vi "UI.KeyCheck.vi"(7 "baud rate (9600)":u32=9600 caption="波特率(9600)", 8 "error in (no error)":errorcluster caption="错误输入（无错误）", 9 "KeyDelay(s)":dbl=8.0 format="%#_2g", 10 "VISA resource name":refnum<visa-resource-name> caption="Serial Port", 11 "KeyList":path) -> (0 "error out":errorcluster caption="错误输出", 3 "Result?":bool, 6 "Test Process":string="Descripte test process.")   [LabVIEW 2012, in "Lib_UEL.ATE.lvlib" / "Lib_App.lvlib"]
uses:
  Lib_App.lvlib
  <vilib>/Utility/config.llb/Read Key (String).vi
  <vilib>/Instr/_visa.llb/VISA Configure Serial Port (Instr).vi
  <vilib>/Utility/config.llb/NI_LVConfig.lvlib
panel:
  in  "para":enum32{"para"}(tab)
  in  "计时":bool
  in  "RS232_ON?":bool
  in  "重置计时":bool=TRUE caption="重置"
  out "KeyCheckOK?":bool[](array[boolean])
  in  "停止":bool
  out "KeyValue":string[](array[string])
  out "Key Frame Check":string
  out "KEY10":bool caption="KEY1"
  out "KEY9":bool caption="KEY1"
  out "KEY8":bool caption="KEY1"
  out "KEY7":bool caption="KEY1"
  out "KEY6":bool caption="KEY1"
  out "KEY5":bool caption="KEY1"
  out "KEY4":bool caption="KEY1"
  out "KEY3":bool caption="KEY1"
  out "KEY2":bool caption="KEY1"
  out "KEY1":bool
  out "KeyTime":dbl format="%05.2f"
  out "Key Frame":string
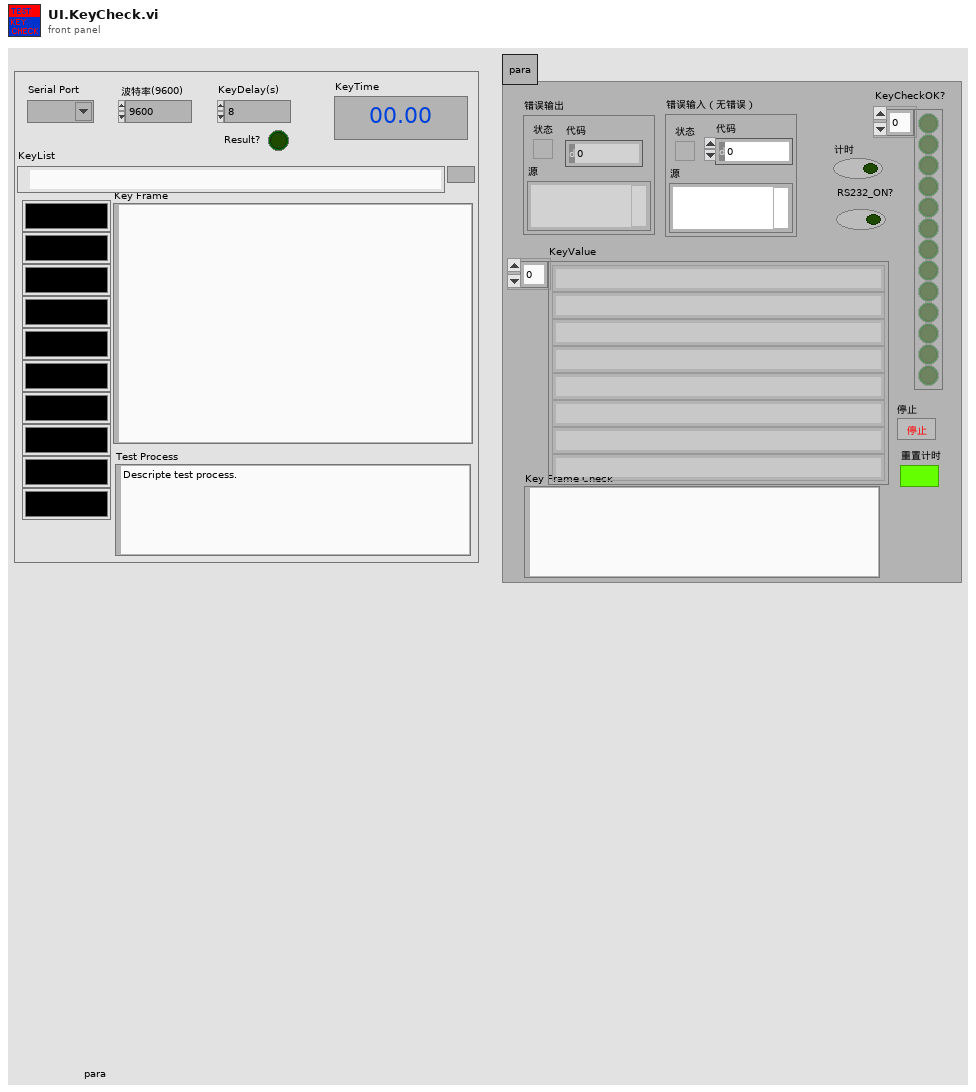
[diagram p1: front panel]
types:
  T1 = typedef "NI_LVConfig.lvlib/Config Data RefNum.ctl" = refnum<k1>
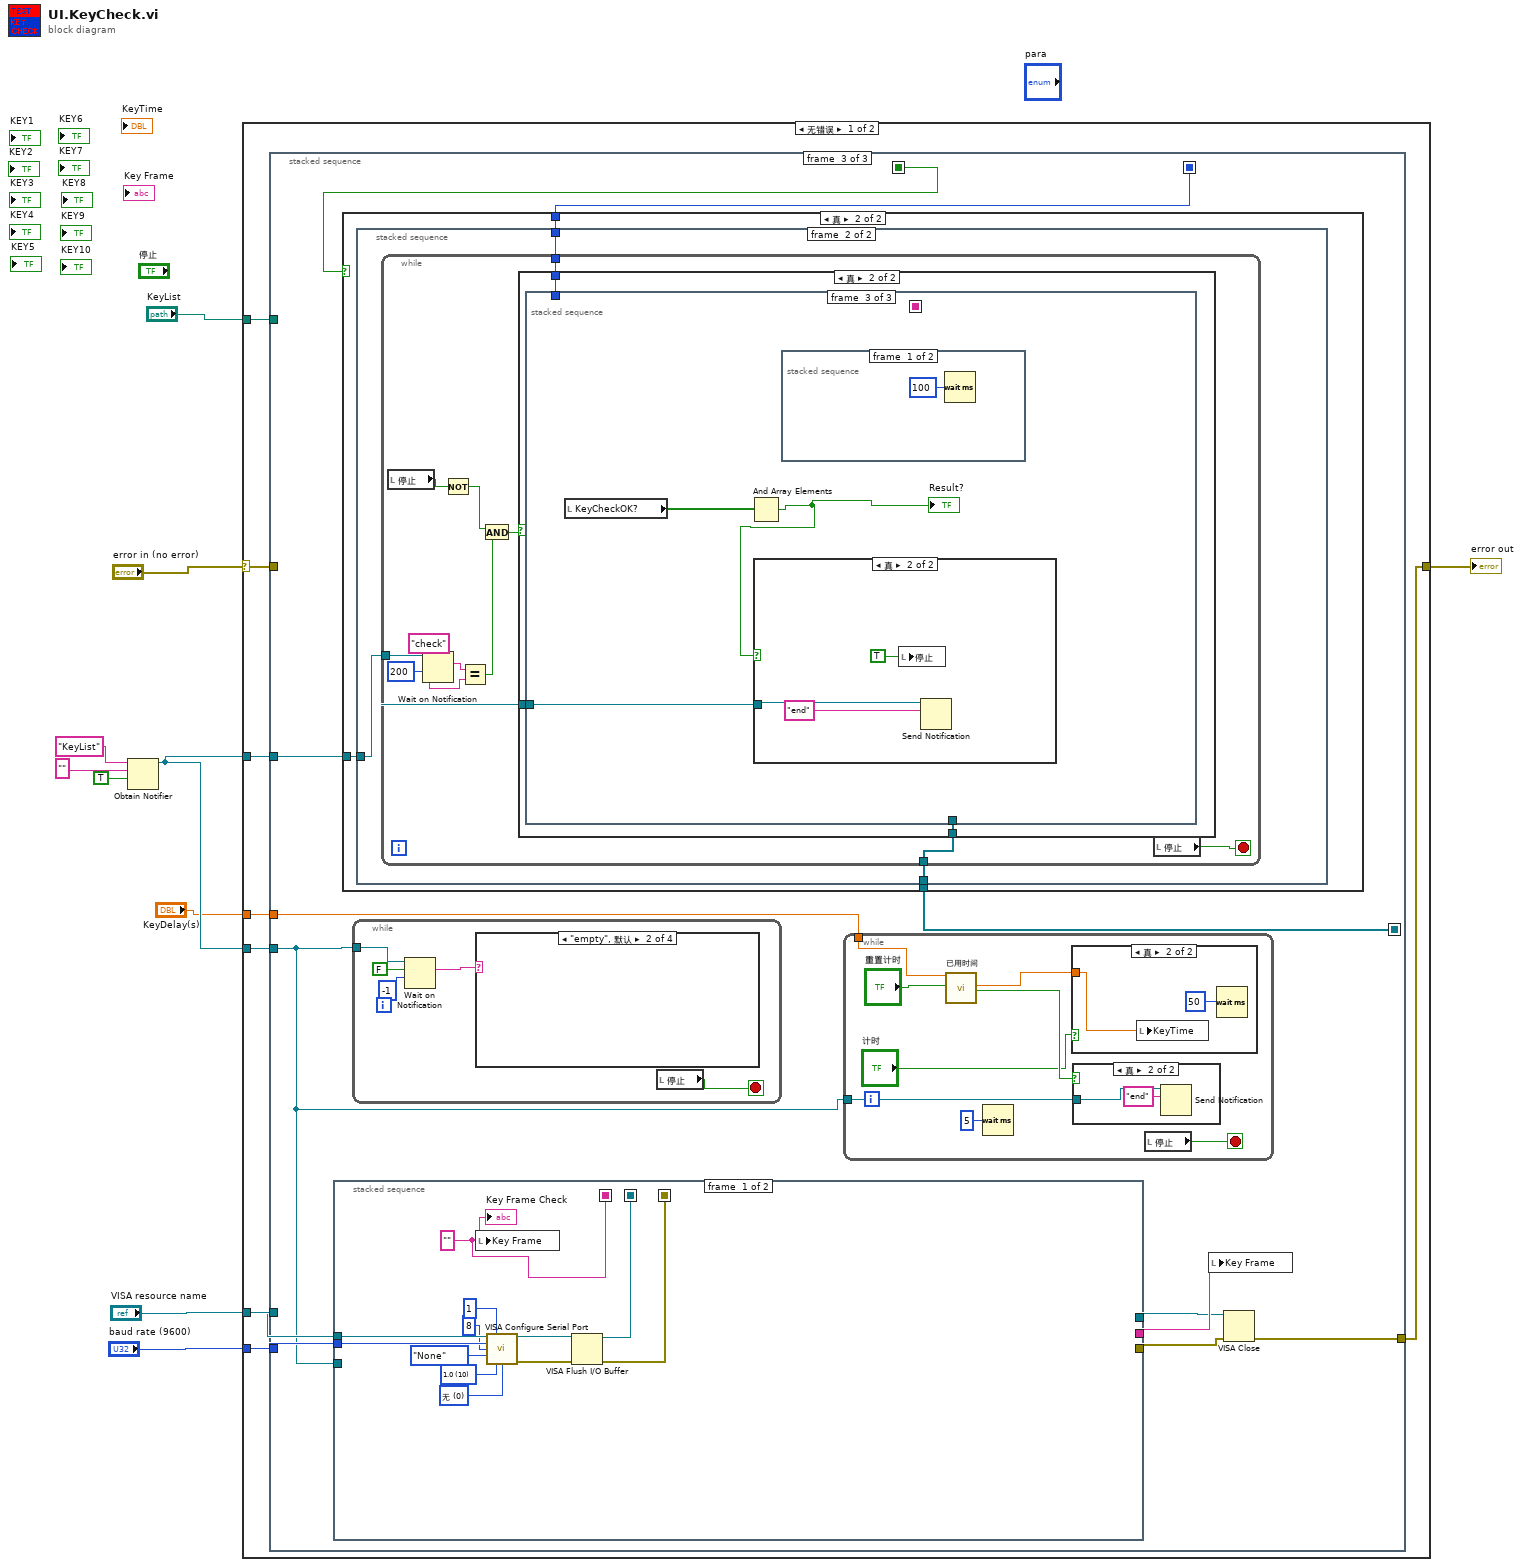
[diagram p0: block diagram]
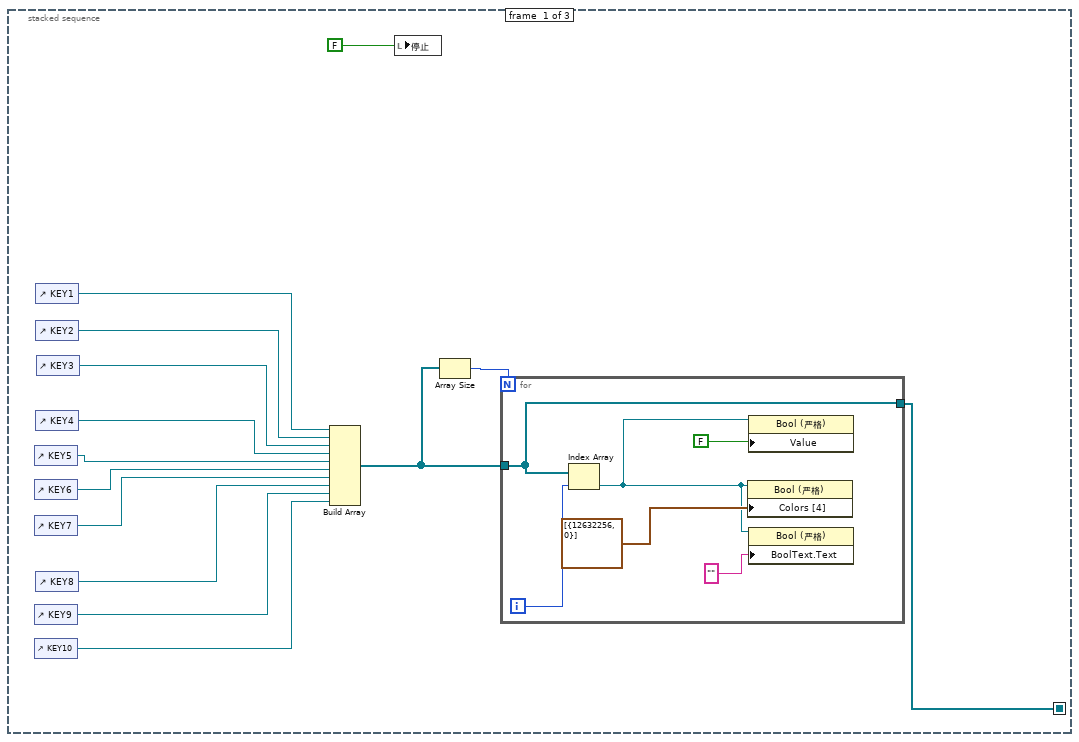
[diagram p2: hidden frame]
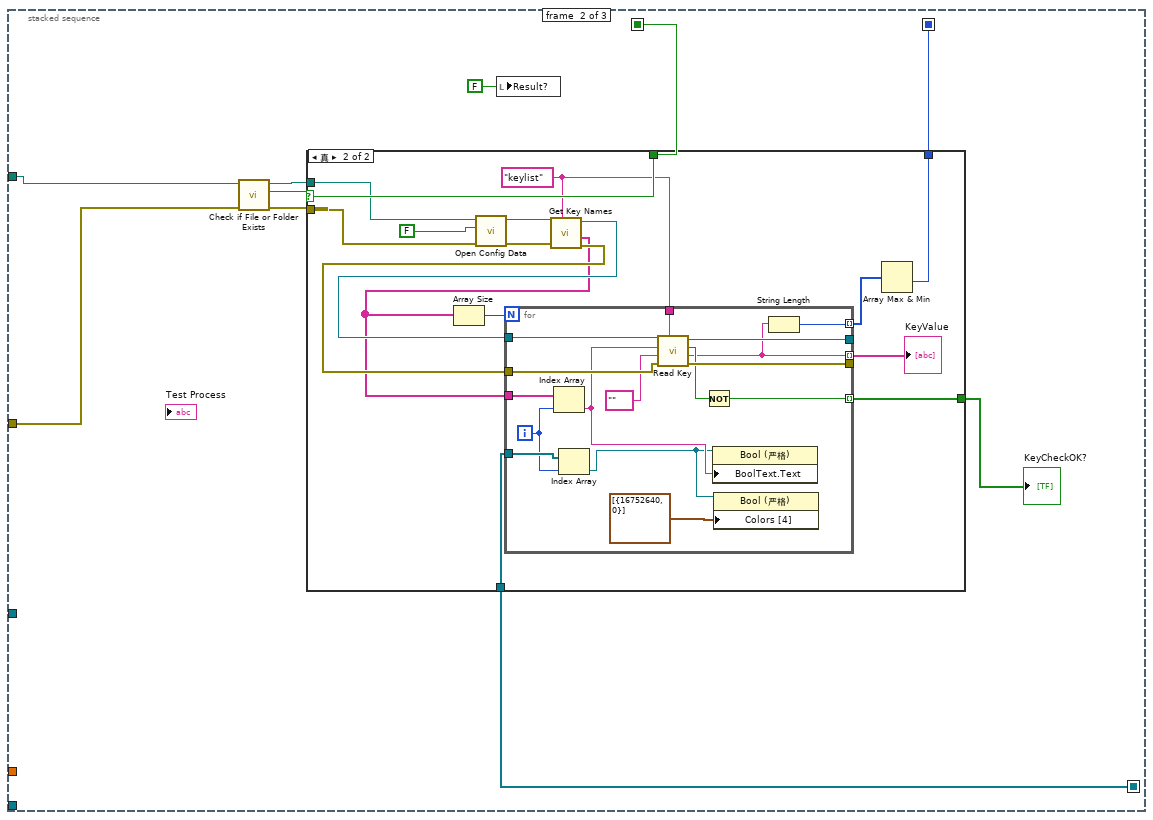
[diagram p3: hidden frame]
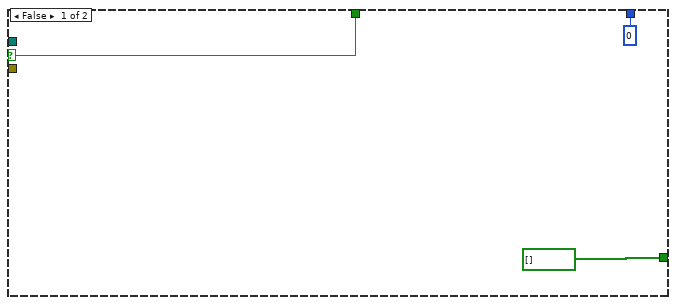
[diagram p4: hidden frame]
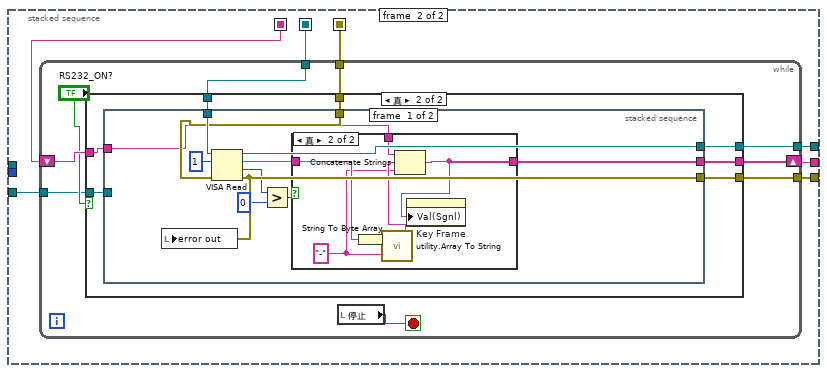
[diagram p5: hidden frame]
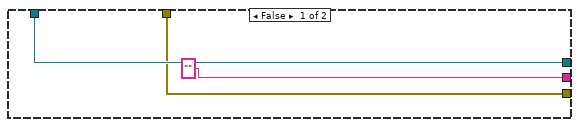
[diagram p6: hidden frame]
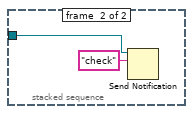
[diagram p8: hidden frame]
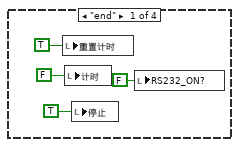
[diagram p11: hidden frame]
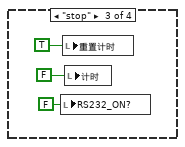
[diagram p12: hidden frame]
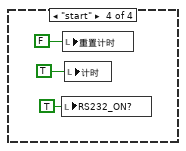
[diagram p13: hidden frame]
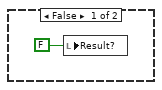
[diagram p14: hidden frame]
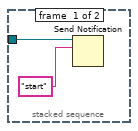
[diagram p15: hidden frame]
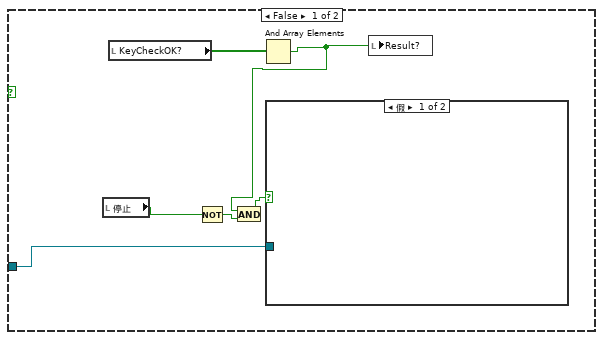
[diagram p16: hidden frame]
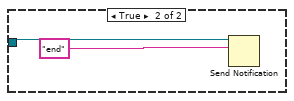
[diagram p17: hidden frame]
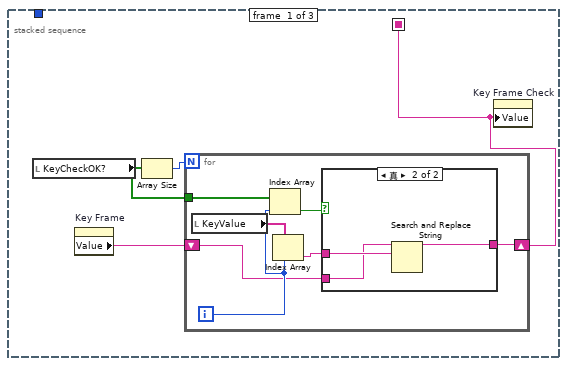
[diagram p18: hidden frame]
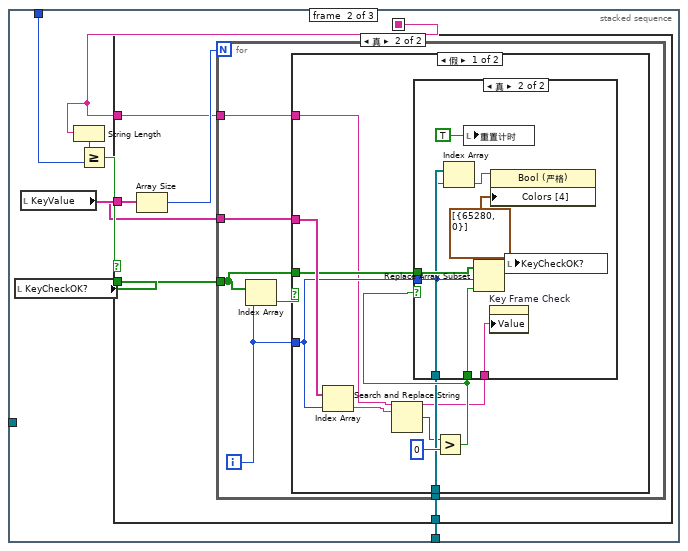
[diagram p20: hidden frame]
diagram:
  n1 = Obtain Notifier(name (unnamed)="KeyList" ("名称（未命名）"), notification data type="" ("名称（未命名）"), create if not found? (T)=TRUE ("如未找到是否创建？(T)")) -> (notifier out=w4:refnum<notifier>)  [unwired: 1 in, 2 out]
  n2 = case shown="无错误" "error in (no error)" {
    selector: "error in (no error)" -> [w17 w272]
    tunnel: [w11 w272] -> w9
    tunnel: "KeyList" -> [w18 _]
    tunnel: w4 -> [w16 _]
    tunnel: w4 -> [w15 _]
    tunnel: "KeyDelay(s)" -> [w14 _]
    tunnel: "VISA resource name" -> [w13 _]
    tunnel: "baud rate (9600)" -> [w12 _]
    frame No Error {
      n3 = stacked-sequence {
        seq-local: [_ w43 _] -> [_ _ w95]
        seq-local: [w28 _ _] -> [_ w42 w93]
        seq-local: [_ w40 _] -> [_ _ w92]
        tunnel: w18 -> [_ w39 _]
        tunnel: w17 -> [_ w44 _]
        tunnel: w16 -> [_ _ w94]
        tunnel: w15 -> [_ _ w85]
        tunnel: w14 -> [_ _ w91]
        tunnel: w13 -> [_ _ w87]
        tunnel: w12 -> [_ _ w86]
        tunnel: [_ _ w84] -> w11
        frame #0 {
          n4 = control-ref of="KEY5"() -> (w25:refnum<vi>)
          n5 = control-ref of="KEY6"() -> (w24:refnum<vi>)
          n6 = control-ref of="KEY7"() -> (w23:refnum<vi>)
          n7 = control-ref of="KEY9"() -> (w21:refnum<vi>)
          n8 = control-ref of="KEY10"() -> (w20:refnum<vi>)
          n9 = control-ref of="KEY1"() -> (w32:refnum<vi>)
          n10 = control-ref of="KEY2"() -> (w31:refnum<vi>)
          n11 = control-ref of="KEY4"() -> (w26:refnum<vi>)
          n12 = control-ref of="KEY8"() -> (w22:refnum<vi>)
          n13 = control-ref of="KEY3"() -> (w27:refnum<vi>)
          n14 = Build Array(w32, w31, w27, w26, w25, w24, w23, w22, w21, w20) -> (w30:refnum<vi>[])
          n15 = local write "停止"(FALSE ("停止")) -> ()
          n16 = Array Size(array=w30) -> (size(s)=w29:i32)
          n17 = for {
            N: w29 -> [_]
            tunnel: w30 -> [w36]
            tunnel: [w36] -> w28
            i -> [w38]
            n18 = Index Array(array=w36, index=w38) -> (element=w34:refnum<vi>)
            n19 = property class="Bool (严格)"(reference=w34, "Colors [4]"=cluster{u32, u32}[] [{12632256, 0}] ("颜色[4]")) -> ()  [unwired: 1 in, 2 out]
            n20 = property class="Bool (严格)"(reference=w34, "Value"=FALSE ("值")) -> ()  [unwired: 1 in, 2 out]
            n21 = property class="Bool (严格)"(reference=w34, "BoolText.Text"="" ("布尔文本.文本")) -> ()  [unwired: 1 in, 2 out]
          }
        }
        frame #1 {
          n22 = call <vilib>:"Check if File or Folder Exists.vi"("error in (no error)"=w44, "path"=w39) -> ("error out"=w46:errorcluster, "file or folder exists?"=w47:bool, "dup path"=w45:path)  [unwired: 7 in]
          n23 = case shown="真" w47 {
            selector: w47 -> [w51 w67]
            tunnel: w46 -> [_ w64]
            tunnel: w45 -> [_ w65]
            tunnel: [w51 w67] -> w43
            tunnel: w42 -> [_ w55]
            tunnel: [bool[] [] w54] -> w41
            tunnel: [0 w52] -> w40
            frame False {
            }
            frame True {
              w58 = "keylist" ("section")
              n24 = call <vilib>:"Open Config Data.vi"("error in (no error)"=w64, "create file if necessary (T)"=FALSE ("create file if necessary? (T)"), "configuration file path"=w65) -> ("error out"=w62:errorcluster, "refnum"=w63:T1)  [unwired: 6 in, 1 out]
              n25 = call <vilib>:"Get Key Names.vi"("section"=w58, "error in (no error)"=w62, "refnum"=w63) -> ("error out"=w59:errorcluster, "key names"=w57:string[], "refnum out"=w60:T1)  [unwired: 5 in, 1 out]
              n26 = Array Size(array=w57) -> (size(s)=w61:i32)
              n27 = for {
                N: w61 -> [_]
                tunnel: w60 -> [w83]
                tunnel: w59 -> [w81]
                tunnel: w58 -> [w82]
                tunnel: w57 -> [w79]
                tunnel: [w78] -> _
                tunnel: [w77] -> _
                tunnel: [w69] -> w56 mode=indexing
                tunnel: w55 -> [w76]
                tunnel: [w70] -> w54 mode=indexing
                tunnel: [w68] -> w53 mode=indexing
                i -> [w75]
                n28 = Index Array(array=w79, index=w75) -> (element=w74:string)
                n29 = Index Array(array=w76, index=w75) -> (element=w73:refnum<vi>)
                n30 = call-poly <vilib>:"Read Key.vi"("section"=w82, "error in (no error)"=w81, "default value"="" ("section"), "key"=w74, "refnum"=w83) -> ("error out"=w77:errorcluster, "value"=w69:string, "found?"=w71:bool, "refnum out"=w78:T1)  [unwired: 3 in]
                n31 = Not(x=w71) -> (.not. x?=w70:bool)
                n32 = property class="Bool (严格)"(reference=w73, "BoolText.Text"=w74) -> ()  [unwired: 1 in, 2 out]
                n33 = property class="Bool (严格)"(reference=w73, "Colors [4]"=cluster{u32, u32}[] [{16752640, 0}] ("颜色[4]")) -> ()  [unwired: 1 in, 2 out]
                n34 = String Length(string=w69) -> (length=w68:i32)
              }
              "KeyValue" <- w56
              n35 = Array Max & Min(array=w53) -> (min value=w52:i32)  [unwired: 3 out]
            }
          }
          "KeyCheckOK?" <- w41
          n36 = local write "Result?"(FALSE ("Result?")) -> ()
        }
        frame #2 {
          n37 = stacked-sequence {
            seq-local: [w103 _] -> [_ w114]
            seq-local: [w102 _] -> [_ w113]
            seq-local: [w96 _] -> [_ w110]
            tunnel: w87 -> [w107 _]
            tunnel: w86 -> [w106 _]
            tunnel: [_ w112] -> w88
            tunnel: [_ w111] -> w89
            tunnel: [_ w109] -> w90
            tunnel: w85 -> [_ w108]
            frame #0 {
              w96 = "" ("名称（未命名）")
              w97 = u16 0 items=["无", "XON/XOFF", "RTS/CTS", "XON/XOFF & RTS/CTS", "DTR/DSR", "XON/XOFF & DTR/DSR"] ("flow control (0:none)")
              w98 = u16 10 items=["1.0"=10, "1.5"=15, "2.0"=20] ("stop bits (10: 1 bit)")
              n38 = local write "Key Frame"(w96) -> ()
              n39 = call-poly "VISA Configure Serial Port"("VISA resource name"=w107, "timeout (10sec)"=u32 1, "baud rate (9600)"=w106, "data bits (8)"=u16 8, "parity (0:none)"=enum16{"None", "Odd", "Even", "Mark", "Space"}."None", "stop bits (10: 1 bit)"=w98, "flow control (0:none)"=w97) -> ("VISA resource name out"=w105:refnum<visa-resource-name>, "error out"=w104:errorcluster)  [unwired: 7 in]
              n40 = VISA Flush I/O Buffer(VISA resource name=w105, error in (no error)=w104) -> (VISA resource name out=w103:refnum<visa-resource-name>, error out=w102:errorcluster)  [unwired: 1 in]
              "Key Frame Check" <- w96
            }
            frame #1 {
              n41 = while {
                tunnel: w114 -> [w122]
                tunnel: w113 -> [w121]
                tunnel: [w120] -> w112
                tunnel: [w119] -> w111
                shift-right: [w117] -> w109
                shift-left: w110 -> [w118]
                tunnel: w108 -> [w115]
                stop <- w123 stop-if-true
                n42 = case shown="真" "RS232_ON?" {
                  tunnel: w122 -> [w126 w133]
                  tunnel: w121 -> [w125 w132]
                  tunnel: [w126 w131] -> w120
                  tunnel: [w125 w130] -> w119
                  tunnel: w118 -> [_ w129]
                  tunnel: ["" w128] -> w117
                  tunnel: w115 -> [_ w127]
                  frame False {
                  }
                  frame True {
                    n43 = stacked-sequence {
                      tunnel: w133 -> [w144 _]
                      tunnel: w132 -> [w143 _]
                      tunnel: [w141 _] -> w131
                      tunnel: [w139 _] -> w130
                      tunnel: w129 -> [w140 _]
                      tunnel: [w138 _] -> w128
                      tunnel: w127 -> [_ w152]
                      frame #0 {
                        n44 = VISA Read(VISA resource name=w144, byte count=u32 1 ("字节总数"), error in (no error)=w143) -> (VISA resource name out=w141:refnum<visa-resource-name>, read buffer=w137:string, return count=w136:u32, error out=w139:errorcluster)
                        n45 = local write "error out"(w139) -> ()
                        n46 = Greater?(x=w136, y=u32 0) -> (0:w134:bool)
                        n47 = case shown="真" w134 {
                          tunnel: w140 -> [w145 w151]
                          tunnel: [w145 w150] -> w138
                          tunnel: w137 -> [_ w149]
                          frame False {
                          }
                          frame True {
                            w146 = "-" ("分隔符输入")
                            n48 = String To Byte Array(string=w149) -> (unsigned byte array=w148:u8[])
                            n49 = call "utility.Array To String.vi"("分隔符输入"=w146, "无符号字节数组"=w148) -> ("命令输出(字符串)"=w147:string)  [unwired: 1 out]
                            n50 = Concatenate Strings(w151, w147, w146) -> (w150:string)
                            n51 = property on="Key Frame" class="Str"("Val(Sgnl)"=w150) -> ()  [unwired: 2 in, 2 out]
                          }
                        }
                      }
                      frame #1 {
                        n52 = Send Notification(notification="check" ("通知"), notifier=w152) -> ()  [unwired: 1 in, 2 out]
                      }
                    }
                  }
                }
                n53 = local read "停止"() -> (w123:bool)
              }
            }
          }
          n54 = case shown="真" w95 {
            tunnel: w94 -> [_ w184]
            tunnel: w93 -> [_ w183]
            tunnel: w92 -> [_ w182]
            frame False {
              n55 = local write "Result?"(FALSE ("Result?")) -> ()
            }
            frame True {
              n56 = stacked-sequence {
                tunnel: w184 -> [w186 w188]
                tunnel: w183 -> [_ w189]
                tunnel: w182 -> [_ w187]
                frame #0 {
                  n57 = Send Notification(notification="start" ("通知"), notifier=w186) -> ()  [unwired: 1 in, 2 out]
                }
                frame #1 {
                  n58 = while {
                    tunnel: w189 -> [w200]
                    tunnel: w188 -> [w197]
                    tunnel: w187 -> [w190]
                    stop <- w196 stop-if-true
                    n59 = local read "停止"() -> (w192:bool)
                    n60 = Wait on Notification(notifier=w197, timeout in ms (-1)=200 ("超时毫秒(-1)")) -> (notification=w199:string)  [unwired: 2 in, 3 out]
                    n61 = Not(x=w192) -> (.not. x?=w191:bool)
                    n62 = Equal?(x=w199, y="check") -> (x = y?=w193:bool)
                    n63 = And(x=w191, y=w193) -> (x .and. y?=w194:bool)
                    n64 = case shown="真" w194 {
                      tunnel: w200 -> [_ w211]
                      tunnel: w197 -> [w205 w210]
                      tunnel: w190 -> [_ w209]
                      frame False {
                        n65 = local read "停止"() -> (w204:bool)
                        n66 = local read "KeyCheckOK?"() -> (w206:bool[])
                        n67 = Not(x=w204) -> (.not. x?=w203:bool)
                        n68 = And Array Elements(Boolean array=w206) -> (logical AND=w202:bool)
                        n69 = And(x=w202, y=w203) -> (x .and. y?=w201:bool)
                        n70 = case shown="假" w201 {
                          tunnel: w205 -> [_ w207]
                          frame False {
                          }
                          frame True {
                            n71 = Send Notification(notification="end" ("通知"), notifier=w207) -> ()  [unwired: 1 in, 2 out]
                          }
                        }
                        n72 = local write "Result?"(w202) -> ()
                      }
                      frame True {
                        n73 = stacked-sequence {
                          seq-local: [w212 _ _] -> [_ w230 _]
                          tunnel: w210 -> [_ _ w265]
                          tunnel: w211 -> [_ w232 _]
                          tunnel: w209 -> [_ w227 _]
                          frame #0 {
                            n74 = local read "KeyCheckOK?"() -> (w214:bool[])
                            n75 = property on="Key Frame" class="Str"() -> ("Value"=w213:string)  [unwired: 2 in, 2 out]
                            n76 = Array Size(array=w214) -> (size(s)=w215:i32)
                            n77 = for {
                              N: w215 -> [_]
                              tunnel: w214 -> [w221]
                              shift-right: [w216] -> w212
                              shift-left: w213 -> [w217]
                              i -> [w220]
                              n78 = local read "KeyValue"() -> (w222:string[])
                              n79 = Index Array(array=w221, index=w220) -> (element=w219:bool)
                              n80 = Index Array(array=w222, index=w220) -> (element=w218:string)
                              n81 = case shown="真" w219 {
                                tunnel: w218 -> [_ w226]
                                tunnel: w217 -> [w223 w225]
                                tunnel: [w223 w224] -> w216
                                frame False {
                                }
                                frame True {
                                n82 = Search and Replace String(input string=w225, search string=w226) -> (result string=w224:string)  [unwired: 6 in, 3 out]
                                }
                              }
                            }
                            n83 = property on="Key Frame Check" class="Str"("Value"=w212) -> ()  [unwired: 2 in, 2 out]
                          }
                          frame #1 {
                            n84 = local read "KeyCheckOK?"() -> (w231:bool[])
                            n85 = local read "KeyValue"() -> (w233:string[])
                            n86 = String Length(string=w230) -> (length=w229:i32)
                            n87 = Greater Or Equal?(x=w229, y=w227) -> (x >= y?=w228:bool)
                            n88 = case shown="真" w228 {
                              tunnel: w233 -> [_ w237]
                              tunnel: w232 -> [_ w236]
                              tunnel: w231 -> [_ w235]
                              tunnel: w230 -> [_ w234]
                              frame False {
                              }
                              frame True {
                                n89 = Array Size(array=w237) -> (size(s)=w238:i32)
                                n90 = for {
                                N: w238 -> [_]
                                tunnel: w235 -> [w241]
                                tunnel: w237 -> [w243]
                                tunnel: w236 -> [w240]
                                tunnel: w234 -> [w239]
                                i -> [w242]
                                n91 = Index Array(array=w241, index=w242) -> (element=w244:bool)
                                n92 = case shown="假" w244 {
                                tunnel: w243 -> [w254 _]
                                tunnel: w242 -> [w251 _]
                                tunnel: w241 -> [w252 _]
                                tunnel: w240 -> [w249 _]
                                tunnel: w239 -> [w248 _]
                                frame False {
                                n93 = Index Array(array=w254, index=w251) -> (element=w245:string)
                                n94 = Search and Replace String(input string=w248, search string=w245) -> (result string=w246:string, number of replacements=w247:i32)  [unwired: 6 in, 2 out]
                                n95 = Greater?(x=w247, y=0) -> (0:w250:bool)
                                n96 = case shown="真" w250 {
                                tunnel: w252 -> [_ w263]
                                tunnel: w251 -> [_ w259]
                                tunnel: w250 -> [_ w262]
                                tunnel: w249 -> [_ w260]
                                tunnel: w246 -> [_ w256]
                                frame False {
                                }
                                frame True {
                                n97 = Index Array(array=w260, index=w259) -> (element=w258:refnum<vi>)
                                n98 = local write "重置计时"(TRUE ("重置计时")) -> ()
                                n99 = Replace Array Subset(array=w263, new element=w262, index=w259) -> (w261:bool[])
                                n100 = property on="Key Frame Check" class="Str"("Value"=w256) -> ()  [unwired: 2 in, 2 out]
                                n101 = property class="Bool (严格)"(reference=w258, "Colors [4]"=cluster{u32, u32}[] [{65280, 0}] ("颜色[4]")) -> ()  [unwired: 1 in, 2 out]
                                n102 = local write "KeyCheckOK?"(w261) -> ()
                                }
                                }
                                }
                                frame True {
                                }
                                }
                                }
                              }
                            }
                          }
                          frame #2 {
                            n103 = local read "KeyCheckOK?"() -> (w266:bool[])
                            n104 = And Array Elements(Boolean array=w266) -> (logical AND=w264:bool)
                            "Result?" <- w264
                            n105 = case shown="真" w264 {
                              tunnel: w265 -> [_ w270]
                              frame False {
                              }
                              frame True {
                                n106 = local write "停止"(TRUE ("停止")) -> ()
                                n107 = Send Notification(notification="end" ("通知"), notifier=w270) -> ()  [unwired: 1 in, 2 out]
                              }
                            }
                            n108 = stacked-sequence {
                              frame #0 {
                                n109 = Wait (ms)(milliseconds to wait=u32 100 ("等待时间（毫秒）")) -> ()  [unwired: 1 out]
                              }
                              frame #1 {
                                n110 = local write "重置计时"(FALSE ("重置计时")) -> ()
                              }
                            }
                          }
                        }
                      }
                    }
                    n111 = local read "停止"() -> (w196:bool)
                  }
                }
              }
            }
          }
          n112 = while {
            tunnel: w85 -> [w170]
            stop <- w167 stop-if-true
            n113 = Wait on Notification(notifier=w170, ignore previous (F)=FALSE ("忽略上一个(F)"), timeout in ms (-1)=-1 ("超时毫秒(-1)")) -> (notification=w168:string)  [unwired: 1 in, 3 out]
            n114 = case shown="\"empty\", 默认" w168 {
              frame "end" {
                n115 = local write "重置计时"(TRUE ("重置计时")) -> ()
                n116 = local write "计时"(FALSE ("计时")) -> ()
                n117 = local write "停止"(TRUE ("停止")) -> ()
                n118 = local write "RS232_ON?"(FALSE ("RS232_ON?")) -> ()
              }
              frame "empty", Default {
              }
              frame "stop" {
                n119 = local write "RS232_ON?"(FALSE ("RS232_ON?")) -> ()
                n120 = local write "重置计时"(TRUE ("重置计时")) -> ()
                n121 = local write "计时"(FALSE ("计时")) -> ()
              }
              frame "start" {
                n122 = local write "RS232_ON?"(TRUE ("RS232_ON?")) -> ()
                n123 = local write "重置计时"(FALSE ("重置计时")) -> ()
                n124 = local write "计时"(TRUE ("计时")) -> ()
              }
            }
            n125 = local read "停止"() -> (w167:bool)
          }
          n126 = while {
            tunnel: w85 -> [w158]
            tunnel: w91 -> [w154]
            stop <- w155 stop-if-true
            n127 = call "已用时间"("Time Target (s)"=w154, "Reset"="重置计时") -> ("Elapsed Time (s)"=w161:dbl, "Time has Elapsed"=w159:bool)  [unwired: 10 in, 6 out]
            n128 = Wait (ms)(milliseconds to wait=u32 5 ("等待时间（毫秒）")) -> ()  [unwired: 1 out]
            n129 = case shown="真" "计时" {
              tunnel: w161 -> [_ w164]
              frame False {
              }
              frame True {
                n130 = local write "KeyTime"(w164) -> ()
                n131 = Wait (ms)(milliseconds to wait=u32 50 ("毫秒倍数")) -> ()  [unwired: 1 out]
              }
            }
            n132 = case shown="真" w159 {
              tunnel: w158 -> [_ w163]
              frame False {
              }
              frame True {
                n133 = Send Notification(notification="end" ("通知"), notifier=w163) -> ()  [unwired: 1 in, 2 out]
              }
            }
            n134 = local read "停止"() -> (w155:bool)
          }
          n135 = local write "Key Frame"(w90) -> ()
          n136 = VISA Close(VISA resource name=w88, error in (no error)=w89) -> (error out=w84:errorcluster)
        }
      }
    }
    frame Error {
    }
  }
  "error out" <- w9
